vi "_PC_D999_UpdStatusDescr.vi"(1 "Switch Enable":bool[](array[boolean]), 2 "Description":refnum<vi>) -> ()   [LabVIEW 2018]
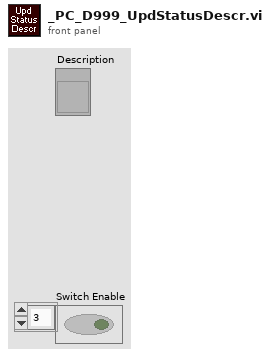
[diagram p1: front panel]
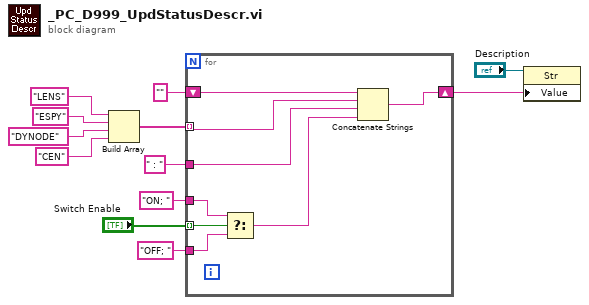
[diagram p0: block diagram]
diagram:
  n1 = Build Array("LENS", "ESPY", "DYNODE", "CEN") -> (w8:string[])
  n2 = for {
    tunnel: w8 -> [w15] mode=indexing
    tunnel: "Switch Enable" -> [w20] mode=indexing
    tunnel: "ON; " -> [w19]
    tunnel: "OFF; " -> [w18]
    tunnel: " : " -> [w14]
    shift-right: [w16] -> w1
    shift-left: "" -> [w17]
    n3 = Select(t=w19, s=w20, f=w18) -> (s? t:f=w13:string)
    n4 = Concatenate Strings(w17, w15, w14, w13) -> (w16:string)
  }
  n5 = property class="Str"(reference="Description", "Value"=w1) -> ()  [unwired: 1 in, 2 out]
